vi "OLA Get Message.vi"() -> (0 "Text":string, 1 "OLA Message Type":T1(ring)=enum."Event=")   [LabVIEW 2009]
panel:
  in  "Timeout ms (-1)":i32=-1
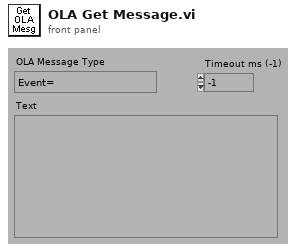
[diagram p1: front panel]
types:
  T1 = enum16{"No Message", "Bad Message", "ClearCharge", "Event=", "Address=", "Ping=", "Stop"}
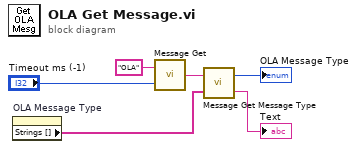
[diagram p0: block diagram]
diagram:
  n1 = property on="OLA Message Type" class="Enum (strict)"() -> ("Strings []"=w3:string[])  [unwired: 2 in, 2 out]
  n2 = call "Message Get.vi"("Timeout ms (-1)"="Timeout ms (-1)", "Module"="OLA") -> ("data out"=w6:string)
  n3 = call "Message Get Message Type.vi"("Message Types"=w3, "Message"=w6) -> ("Trailing text"=→"Text":string, "Message Type"=→"OLA Message Type":i32)
